vi "Begin.vi"(8 "error in":errorcluster) -> (0 "error out":errorcluster, 1 "ADI IMU DevRef":T1={"DevStatus"={"status"=FALSE, "code"=0, "source"=""}, "Handle"=0, "SPI Bus"=enum."SPI On-Board, CS0", "Device Found"=FALSE, "Device Ready"=FALSE, "Yaw Axis"=enum."Z", "AHRS Algorithm"=enum."Complementary", "Serial"=0, "Lot ID 2"=0, "Lot ID 1"=0, "Bytes Per Sample"=0, "Calibrate On Open?"=FALSE}, 2 "JoystickDevRef":T3={"Device"=enum."USB 1"})   [LabVIEW 2018]
doc: "Called before other user functions, this VI can be used to open I/O refnums, load in file data, and do general program initialization. Notice that the <B>error out</B> terminal is simply used for data flow. Wiring it to other structures or subVIs ensures that this VI runs first."
uses:
  <vilib>/Rock Robotics/WPI/Joystick/WPI_JoystickDevRef.ctl
  <vilib>/Rock Robotics/WPI/Joystick/WPI_JoystickDeviceEnum.ctl
  ADIS16448 IMU/ADI_IMU_ADIS16448_IMUDevRef.ctl
  <vilib>/Rock Robotics/SystemInterfaces/spilib/spi_bus.ctl
  <vilib>/Rock Robotics/WPI/DriverStation/WPI_DriverStationRobotMode2.ctl
  Robot Global Data.vi
  <vilib>/Rock Robotics/Network Tables/NT Write String Array.vi
  <vilib>/Rock Robotics/Network Tables/NT Write String.vi
  ADIS16448 IMU/ADIS16448_IMU.lvlib
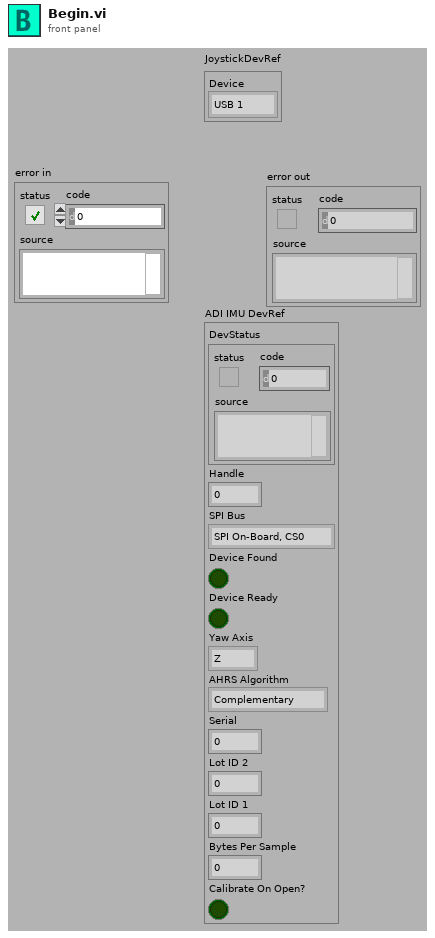
[diagram p1: front panel]
types:
  T1 = typedef "ADIS16448_IMU.lvlib/ADI_IMU_ADIS16448_IMUDevRef.ctl" = cluster{"DevStatus":errorcluster, "Handle":i32, "SPI Bus":T2, "Device Found":bool, "Device Ready":bool, "Yaw Axis":enum16{"X", "Y", "Z"}, "AHRS Algorithm":enum16{"Complementary", "Madgwick"}, "Serial":u16, "Lot ID 2":u16, "Lot ID 1":u16, "Bytes Per Sample":u16, "Calibrate On Open?":bool}
  T2 = typedef "spi_bus.ctl" = enum16{"SPI On-Board, CS0", "SPI On-Board, CS1", "SPI On-Board, CS2", "SPI On-Board, CS3", "SPI MXP", "Invalid"}
  T3 = typedef "WPI_JoystickDevRef.ctl" = cluster{"Device":T4}
  T4 = typedef "WPI_JoystickDeviceEnum.ctl" = enum16{"USB 0", "USB 1", "USB 2", "USB 3", "USB 4", "USB 5"}
  T5 = typedef "WPI_DriverStationRobotMode2.ctl" = enum16{"Autonomous Disabled", "Autonomous Enabled", "Teleop Disabled", "Teleop Enabled", "Disconnected", "Finish", "Test Disabled", "Test Enabled", "Emergency Stopped"}
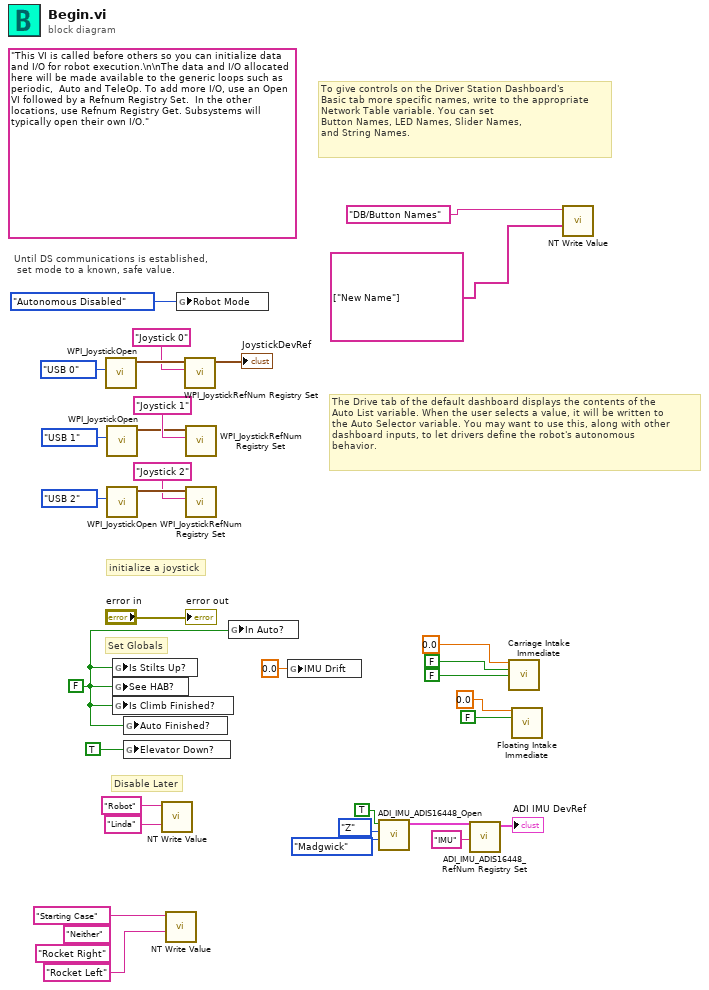
[diagram p0: block diagram]
diagram:
  (unwired) "Rocket Right" ("x")
  (unwired) "Neither" ("String")
  w9 = FALSE ("Is Stilts Up?")
  (unwired) "This VI is called before others so you can initialize data and I/O for robot execution.\n\nThe data and I/O allocated here will be made available to the generic loops such as periodic,  Auto and TeleOp. To add more I/O, use an Open VI followed by a Refnum Registry Set.  In the other locations, use Refnum Registry Get. Subsystems will typically open their own I/O."
  # "Disable Later"
  # "Set Globals"
  # "The Drive tab of the default dashboard displays the contents of the\nAuto List variable. When the user selects a value, it will be written to\nthe Auto Selector variable. You may want to use this, along with other\ndashboard inputs, to let drivers define the robot's autonomous\nbehavior."
  # "To give controls on the Driver Station Dashboard's\nBasic tab more specific names, write to the appropriate\nNetwork Table variable. You can set\nButton Names, LED Names, Slider Names,\nand String Names."
  # "initialize a joystick"
  # "Until DS communications is established,\n set mode to a known, safe value."
  n1 = call <vilib>:"WPI_JoystickOpen.vi"("JoystickDevice"=WPI_JoystickDeviceEnum."USB 0") -> ("JoystickDevRef"=w24:T3)  [unwired: 10 in]
  n2 = call <vilib>:"WPI_JoystickOpen.vi"("JoystickDevice"=WPI_JoystickDeviceEnum."USB 1") -> ("JoystickDevRef"=w30:T3)  [unwired: 10 in]
  n3 = call <vilib>:"WPI_JoystickOpen.vi"("JoystickDevice"=WPI_JoystickDeviceEnum."USB 2") -> ("JoystickDevRef"=w12:T3)  [unwired: 10 in]
  n4 = global write "Robot Global Data.vi" "Is Stilts Up?"(w9) -> ()
  n5 = global write "Robot Global Data.vi" "See HAB?"(w9) -> ()
  n6 = global write "Robot Global Data.vi" "Is Climb Finished?"(w9) -> ()
  n7 = global write "Robot Global Data.vi" "Auto Finished?"(w9) -> ()
  n8 = global write "Robot Global Data.vi" "Elevator Down?"(TRUE ("Auto Finished?")) -> ()
  n9 = call-poly <vilib>:"NT Write Value.vi"("String"="Linda", "Name"="Robot") -> ()  [unwired: 9 in, 1 out]
  n10 = call-poly <vilib>:"NT Write Value.vi"("String"="Rocket Left" ("y"), "Name"="Starting Case") -> ()  [unwired: 9 in, 1 out]
  n11 = global write "Robot Global Data.vi" "Robot Mode"(WPI_DriverStationRobotMode2."Autonomous Disabled" ("Robot Mode")) -> ()
  n12 = call <vilib>:"WPI_JoystickRefNum Registry Set.vi"("refnum name"="Joystick 0", "JoystickDevRef"=w24) -> ("JoystickDevRef"=→"JoystickDevRef":T3)  [unwired: 8 in, 1 out]
  n13 = call <vilib>:"WPI_JoystickRefNum Registry Set.vi"("refnum name"="Joystick 1", "JoystickDevRef"=w30) -> ()  [unwired: 8 in, 2 out]
  n14 = call <vilib>:"WPI_JoystickRefNum Registry Set.vi"("refnum name"="Joystick 2", "JoystickDevRef"=w12) -> ()  [unwired: 8 in, 2 out]
  n15 = global write "Robot Global Data.vi" "In Auto?"(w9) -> ()
  n16 = global write "Robot Global Data.vi" "IMU Drift"(0.0 ("IMU Drift")) -> ()
  n17 = call "ADI_IMU_ADIS16448_Open.vi"("AHRS Algorithm"=enum16{"Complementary", "Madgwick"}."Madgwick", "Yaw Axis"=enum16{"X", "Y", "Z"}."Z", "Calibrate On Open"=TRUE) -> ("ADI IMU DevRef Out"=w3:T1)  [unwired: 7 in, 1 out]
  n18 = call "ADI_IMU_ADIS16448_RefNum Registry Set.vi"("refnum name"="IMU", "ADI IMU DevRef"=w3) -> ("ADI IMU DevRef"=→"ADI IMU DevRef":T1)  [unwired: 8 in, 1 out]
  n19 = call "Carriage Intake Immediate.vi"("Setpoint Left"=0.0 ("Setpoint"), "Extend"=FALSE, "Open"=FALSE ("Grab")) -> ()  [unwired: 12 in, 1 out]
  n20 = call "Floating Intake Immediate.vi"("Setpoint"=0.0, "Switch"=FALSE ("extend")) -> ()  [unwired: 13 in, 1 out]
  n21 = call-poly <vilib>:"NT Write Value.vi"("String Array"=string[] ["New Name"], "Name"="DB/Button Names") -> ()  [unwired: 9 in, 1 out]
  "error out" <- "error in"
